vi "HXG2_PlotInitialize.vi"(7 "Waveform Chart Ref":refnum<vi>, 8 "error in (no error)":errorcluster) -> (0 "error out":errorcluster)   [LabVIEW 2012]
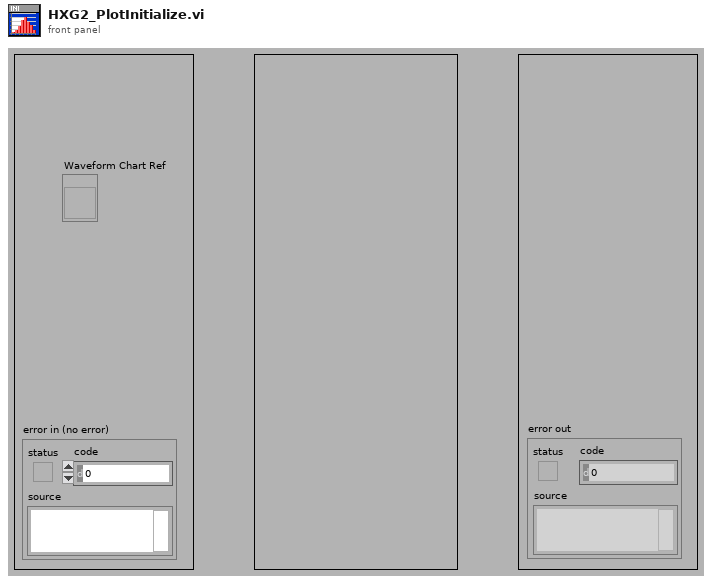
[diagram p1: front panel]
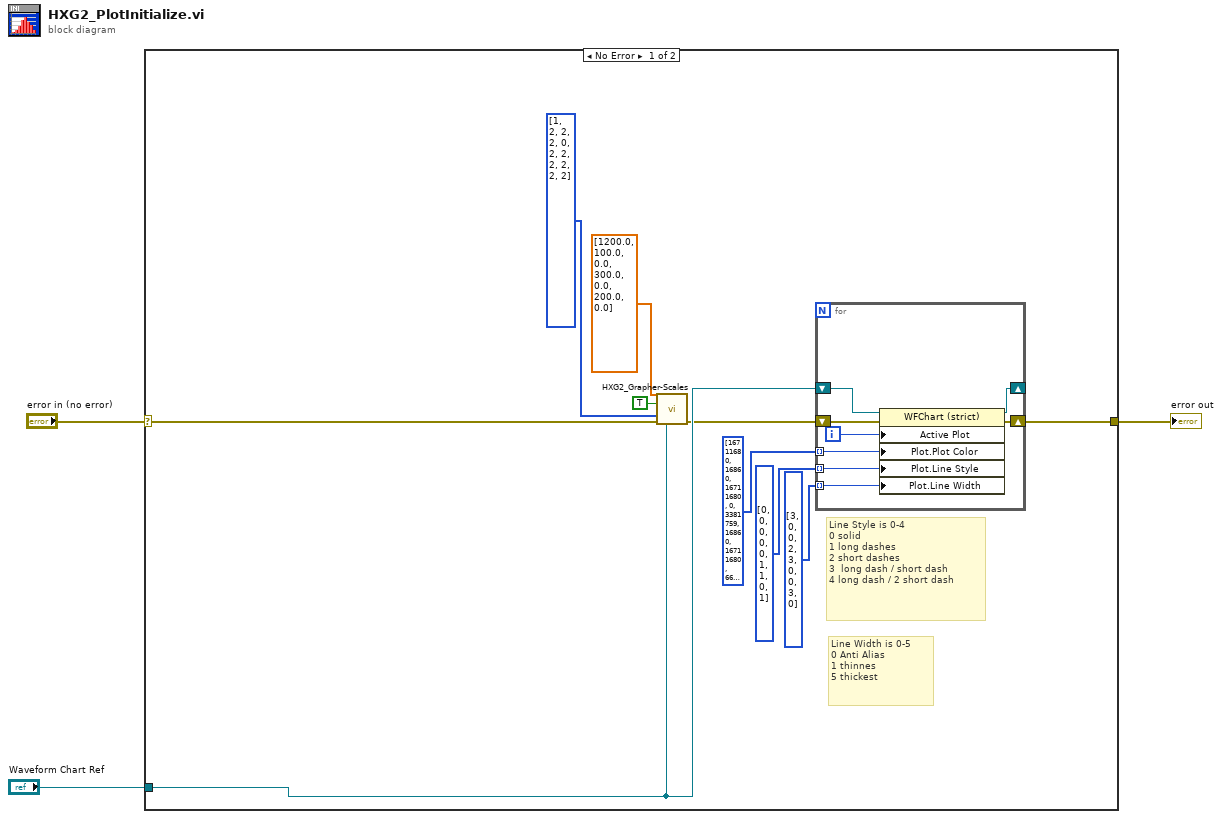
[diagram p0: block diagram]
diagram:
  n1 = case shown="No Error" "error in (no error)" {
    selector: "error in (no error)" -> [w4 w22]
    tunnel: [w8 w22] -> w3
    tunnel: "Waveform Chart Ref" -> [w10 _]
    frame No Error {
      w12 = u32[] [1, 2, 2, 2, 0, 2, 2, 2, 2, 2, 2] items=["1", "2", "3"] ("Graph Scales")
      # "Line Width is 0-5 \n0 Anti Alias\n1 thinnes\n5 thickest"
      # "Line Style is 0-4 \n0 solid\n1 long dashes\n2 short dashes\n3  long dash / short dash\n4 long dash / 2 short dash"
      n2 = call "HXG2_Grapher-Scales.vi"("Graph Scales In"=dbl[] [1200.0, 100.0, 0.0, 300.0, 0.0, 200.0, 0.0], "Update Chart"=TRUE, "Scale Ctrl"=w12, "error in (no error)"=w4, "Waveform Chart Ref in"=w10) -> ("error out"=w9:errorcluster)  [unwired: 10 in]
      n3 = for {
        shift-right: [w19] -> w8
        shift-left: w9 -> [w20]
        tunnel: u32[] [16711680, 16860, 16711680, 0, 3381759, 16860, 16711680, 6618880, 6618880] -> [w17] mode=indexing
        tunnel: u8[] [0, 0, 0, 0, 0, 1, 1, 0, 1] -> [w16] mode=indexing
        tunnel: u8[] [3, 0, 0, 2, 3, 0, 0, 3, 0] -> [w15] mode=indexing
        shift-right: [w14] -> _
        shift-left: w10 -> [w21]
        i -> [w18]
        n4 = property class="WFChart (strict)"(reference=w21, error in=w20, "Active Plot"=w18, "Plot.Plot Color"=w17, "Plot.Line Style"=w16, "Plot.Line Width"=w15) -> (reference out=w14:refnum<vi>, error out=w19:errorcluster)
      }
    }
    frame Error {
    }
  }
  "error out" <- w3
